vi "set_stop.vi"(0 "HGF_Agent.lvclass in":refnum<class "MoAgSy_AgentBase.lvclass">, 5 "error in (no error)":errorcluster, 6 "MoAgSy_Visitor_stop in":refnum<class "MoAgSy_Visitor_stop.lvclass">) -> (14 "HGF_Agent.lvclass out":refnum<class "MoAgSy_AgentBase.lvclass">, 19 "error out":errorcluster)   [LabVIEW 2009, in "MoAgSy_Base.lvlib" / "MoAgSy_AgentBase.lvclass"]
uses:
  MoAgSy_AgentBase.lvclass
  Visitors/MoAgSy_Visitor_stop/MoAgSy_Visitor_stop.lvclass
  MoAgSy_AgentBase.lvclass/MoAgSy_AgentBase.ctl
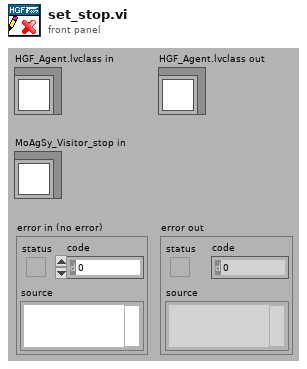
[diagram p1: front panel]
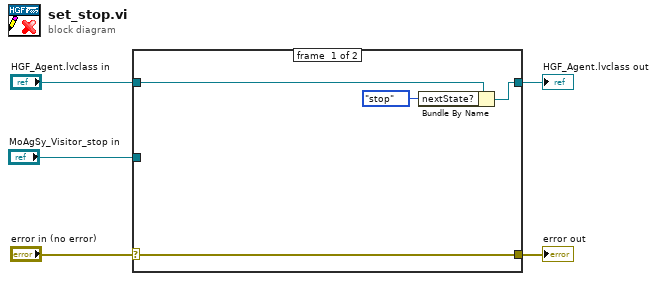
[diagram p0: block diagram]
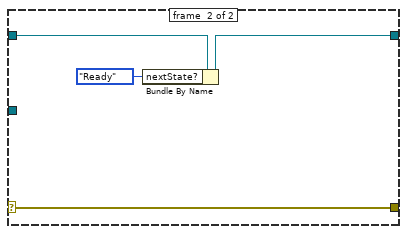
[diagram p2: hidden frame]
diagram:
  n1 = case shown="No Error" "error in (no error)" {
    selector: "error in (no error)" -> [w9 w12]
    tunnel: [w9 w12] -> w4
    tunnel: [w7 w11] -> w2
    tunnel: "HGF_Agent.lvclass in" -> [w8 w13]
    tunnel: "MoAgSy_Visitor_stop in" -> [_ _]
    frame #0 {
      n2 = Bundle By Name(cluster=w8, "nextState?"=enum16{"Ready", "stop", "travel"}."stop") -> (w7:refnum<class "MoAgSy_AgentBase.lvclass">)
    }
    frame #1 {
      n3 = Bundle By Name(cluster=w13, "nextState?"=enum16{"Ready", "stop", "travel"}."Ready") -> (w11:refnum<class "MoAgSy_AgentBase.lvclass">)
    }
  }
  "error out" <- w4
  "HGF_Agent.lvclass out" <- w2
